vi "String_TO_CAN_Frame.vi"(11 "CAN_Frame":string) -> (2 "CAN_FRAME":T1, 3 "DATA_LEN":i32)   [LabVIEW 2020, in "ZLG_CAN.lvlib"]
uses:
  ZLG_CAN.lvlib
  CAN_Frame.ctl
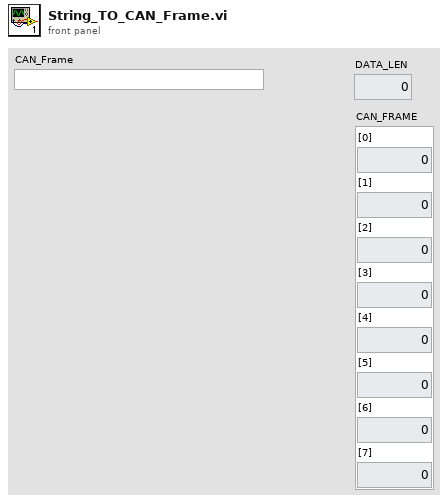
[diagram p1: front panel]
types:
  T1 = typedef "ZLG_CAN.lvlib/CAN_Frame.ctl" = cluster{"[0]":u8, "[1]":u8, "[2]":u8, "[3]":u8, "[4]":u8, "[5]":u8, "[6]":u8, "[7]":u8}
  T2 = cluster{"[0]":u32, "[1]":u32, "[2]":u32, "[3]":u32, "[4]":u32, "[5]":u32, "[6]":u32, "[7]":u32}
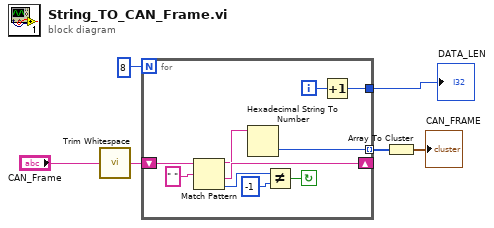
[diagram p0: block diagram]
diagram:
  n1 = call <vilib>:"Trim Whitespace.vi"("string"="CAN_Frame") -> ("trimmed string"=w3:string)  [unwired: 1 in]
  n2 = for {
    N: 8 -> [_]
    shift-right: [w15] -> _
    shift-left: w3 -> [w16]
    tunnel: [w7] -> w5
    tunnel: [w9] -> w2 mode=indexing
    i -> [w11]
    stop <- w8 continue-if-true
    n3 = Match Pattern(string=w16, regular expression=" " ("正则表达式")) -> (before substring=w10:string, after substring=w15:string, offset past match=w13:i32)  [unwired: 1 in, 1 out]
    n4 = Hexadecimal String To Number(string=w10) -> (number=w9:u32)  [unwired: 2 in, 1 out]
    n5 = Not Equal?(x=w13, y=-1) -> (x != y?=w8:bool)
    n6 = Increment(x=w11) -> (x+1=w7:i32)
  }
  "DATA_LEN" <- w5
  n7 = Array To Cluster(array=w2) -> (cluster=→"CAN_FRAME":T2)
